vi "Write supported actions list VI.vi"(8 "error in (no error)":errorcluster, 10 "supported actions list VI":path, 11 "Simple Sequencer TBM configuration in":refnum<class "Simple Sequencer TBM configuration.lvclass">) -> (0 "error out":errorcluster, 3 "Simple Sequencer TBM configuration out":refnum<class "Simple Sequencer TBM configuration.lvclass">)   [LabVIEW 2014, in "Simple Sequencer TBM configuration.lvclass"]
uses:
  Simple Sequencer TBM configuration.lvclass
  Simple Sequencer TBM configuration.lvclass/Simple Sequencer TBM configuration.ctl
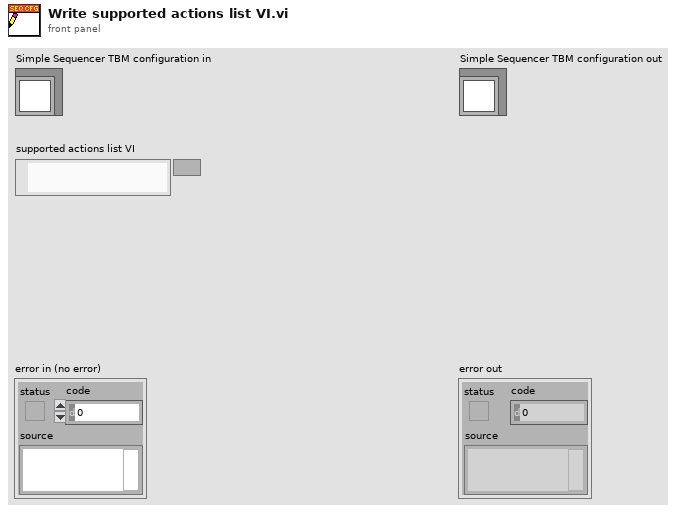
[diagram p1: front panel]
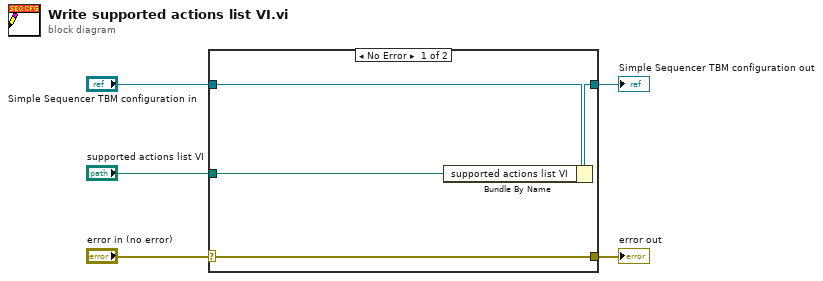
[diagram p0: block diagram]
diagram:
  n1 = case shown="No Error" "error in (no error)" {
    selector: "error in (no error)" -> [w9 w10]
    tunnel: [w9 w10] -> w4
    tunnel: [w7 w11] -> w2
    tunnel: "Simple Sequencer TBM configuration in" -> [w8 w11]
    tunnel: "supported actions list VI" -> [w6 _]
    frame No Error {
      n2 = Bundle By Name(cluster=w8, "supported actions list VI"=w6) -> (w7:refnum<class "Simple Sequencer TBM configuration.lvclass">)
    }
    frame Error {
    }
  }
  "error out" <- w4
  "Simple Sequencer TBM configuration out" <- w2
